vi "Vision Processing.vi"(7 "Image Size":T5=enum."320x240", 8 "error in (no error)":errorcluster, 11 "input cluster":T4={"Image Cal"="remote image 0000000011172DF4", "CameraDevRef"={"Camera Address"="USB 0", "CameraStatus"={"status"=FALSE, "code"=0, "source"=""}}, "Color"="remote image 000000001117C1BC", "Mask"="remote image 000000001106BF6C"}) -> ()   [LabVIEW 2016]
uses:
  Vision Support Code/Camera Types.ctl
  <vilib>/Rock Robotics/WPI/Camera/WPI_CameraImageSize.ctl
  <vilib>/vision/Image Controls.llb/IMAQ Image.ctl
  <vilib>/Rock Robotics/WPI/Camera/WPI_CameraDevRef.ctl
  Robot Global Data.vi
  <vilib>/Rock Robotics/Network Tables/NT Read Number.vi
  <vilib>/Rock Robotics/Network Tables/NT Read String.vi
  Vision Global.vi
  <vilib>/Rock Robotics/Network Tables/NT Write Number.vi
  <vilib>/Rock Robotics/Network Tables/NT Write String.vi
  <vilib>/vision/NI_Vision_Development_Module.lvlib
panel:
  out "LED Color":T1={"Hue"={30.0, 150.0}, "Sat"={0.0, 255.0}, "Val"={121.42857142857143, 255.0}} {"Hue" scale=0.0..255.0 scale format="%#_3g"}
  out "Size Limit %":dbl=0.04 format="%#_13g"
  out "Image":T2(plugin-control)
  out "error out":errorcluster
  out "loop ms":u32=37
  out "Calibration error":errorcluster
  in  "Display Original":bool=TRUE
  in  "Display Mask":bool=TRUE
  in  "Line Border":cluster{"Top":dbl, "Bottom":dbl}={"Top"=6.0, "Bottom"=1.0}
  in  "Use Calibration":bool
  in  "Color Mode":u16(ring)=3 items=["RGB", "HSL", "HSV", "HSI"]
  in  "Particles":dbl=2.0
  in  "Score Cutoff %":dbl=82.0
  in  "Camera Type":T6=enum."MS HD3000 square"
  out "Results":T7={"Distance (ft)"=0.0, "Score"=0.0, "Normalized"={"Center"={-1.0, 1.0}, "Rectangle"={"Numeric"=-1.0, "Numeric 2"=1.0, "Numeric 3"=-1.0, "Numeric 5"=1.0}}, "Pixels"={"Center"={0.0, 0.0}, "Rectangle"={"Numeric"=0.0, "Numeric 2"=0.0, "Numeric 3"=0.0, "Numeric 5"=0.0}}} {"Score" format="%#_3g"; "Pixels"."Rectangle"."Numeric 5" format="%#_3g"; "Pixels"."Rectangle"."Numeric 3" format="%#_3g"; "Pixels"."Rectangle"."Numeric 2" format="%#_3g"; "Pixels"."Rectangle"."Numeric" format="%#_3g"; "Normalized"."Rectangle"."Numeric 5" format="%#_2g"; "Normalized"."Rectangle"."Numeric 3" format="%#_2g"; "Normalized"."Rectangle"."Numeric 2" format="%#_2g"; "Normalized"."Rectangle"."Numeric" format="%#_2g"; "Normalized"."Center"."?" format="%#_3g"; "Normalized"."Center"."?" format="%#_3g"; "Distance (ft)" format="%#_3g"}
  out "Qualified Particles":i32
  # "This is now indicator"
  # "Legend:\n    Rectangle\n       Green - Good target, distance ft\n       Red - Bad target\n    Orange Text - Score in %"
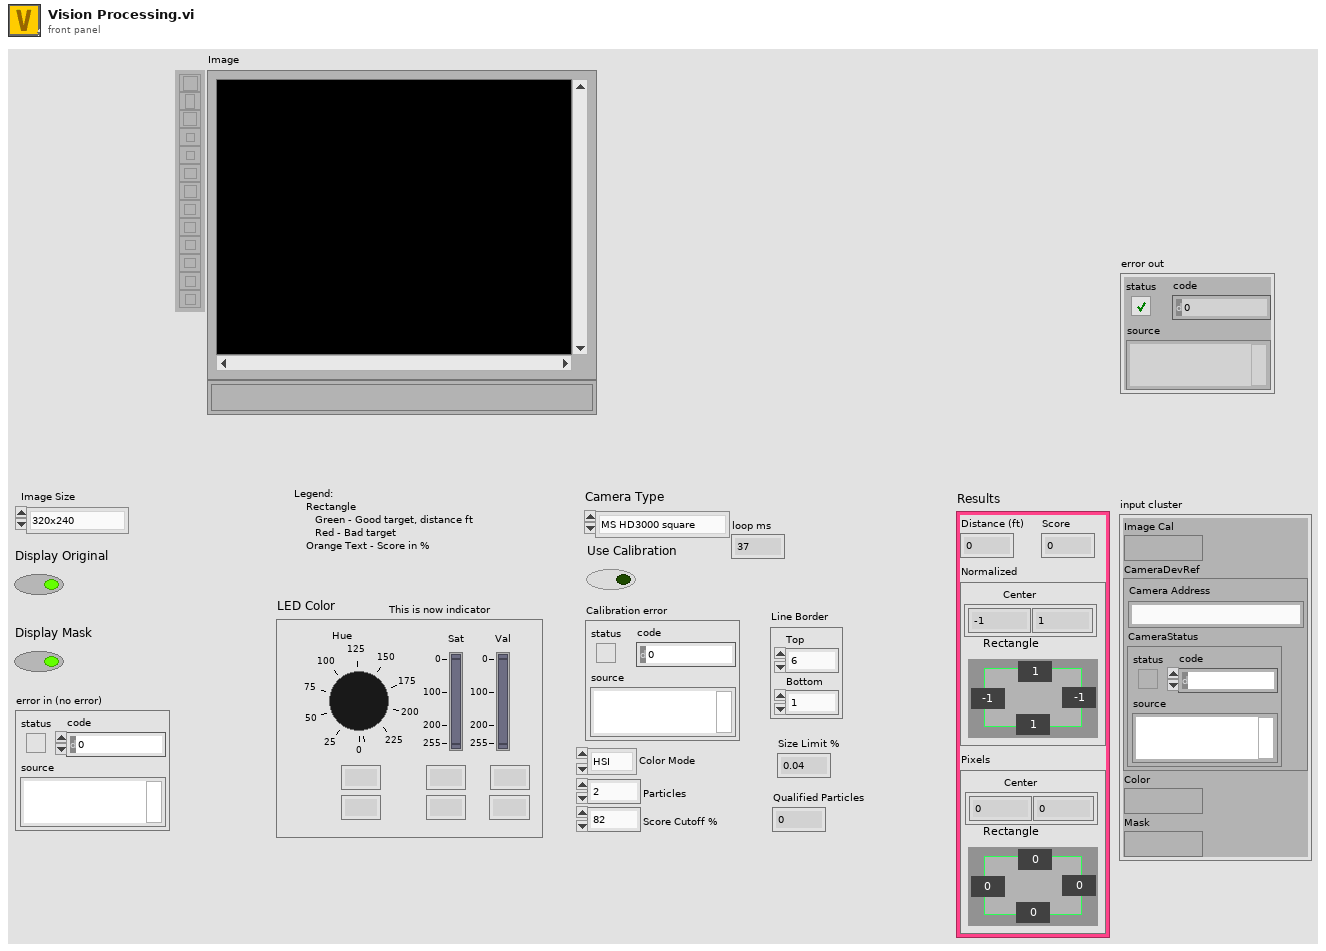
[diagram p1: front panel]
types:
  T1 = cluster{"Hue":cluster{dbl, dbl}, "Sat":cluster{dbl, dbl}, "Val":cluster{dbl, dbl}}
  T2 = typedef "IMAQ Image.ctl" = refnum<image>
  T3 = typedef "WPI_CameraDevRef.ctl" = cluster{"Camera Address":string, "CameraStatus":errorcluster}
  T4 = cluster{"Image Cal":T2, "CameraDevRef":T3, "Color":T2, "Mask":T2}
  T5 = typedef "WPI_CameraImageSize.ctl" = enum16{"640x480", "320x240", "160x120", "Custom"}
  T6 = typedef "Camera Types.ctl" = enum16{"206", "1011", "1013", "MS HD3000 square", "MS HD3000 640x480"}
  T7 = cluster{"Distance (ft)":dbl, "Score":dbl, "Normalized":cluster{"Center":cluster{dbl, dbl}, "Rectangle":cluster{"Numeric":dbl, "Numeric 2":dbl, "Numeric 3":dbl, "Numeric 5":dbl}}, "Pixels":cluster{"Center":cluster{dbl, dbl}, "Rectangle":cluster{"Numeric":dbl, "Numeric 2":dbl, "Numeric 3":dbl, "Numeric 5":dbl}}}
  T8 = typedef "Particle Parameters" = i32
  T9 = cluster{"Left":dbl, "Top":dbl, "Right":dbl, "Bottom":dbl}
  T10 = cluster{"Image out":T2, "Results":cluster{"Distance (ft)":dbl, "Score":dbl, "Normalized":cluster{"Center":cluster{dbl, dbl}, "Rectangle":cluster{"Numeric":dbl, "Numeric 2":dbl, "Numeric 3":dbl, "Numeric 5":dbl}}, "Pixels":cluster{"Center":cluster{dbl, dbl}, "Rectangle":cluster{"Numeric":dbl, "Numeric 2":dbl, "Numeric 3":dbl, "Numeric 5":dbl}}}, "Edges":cluster{"X":sgl, "Y":sgl}[]}
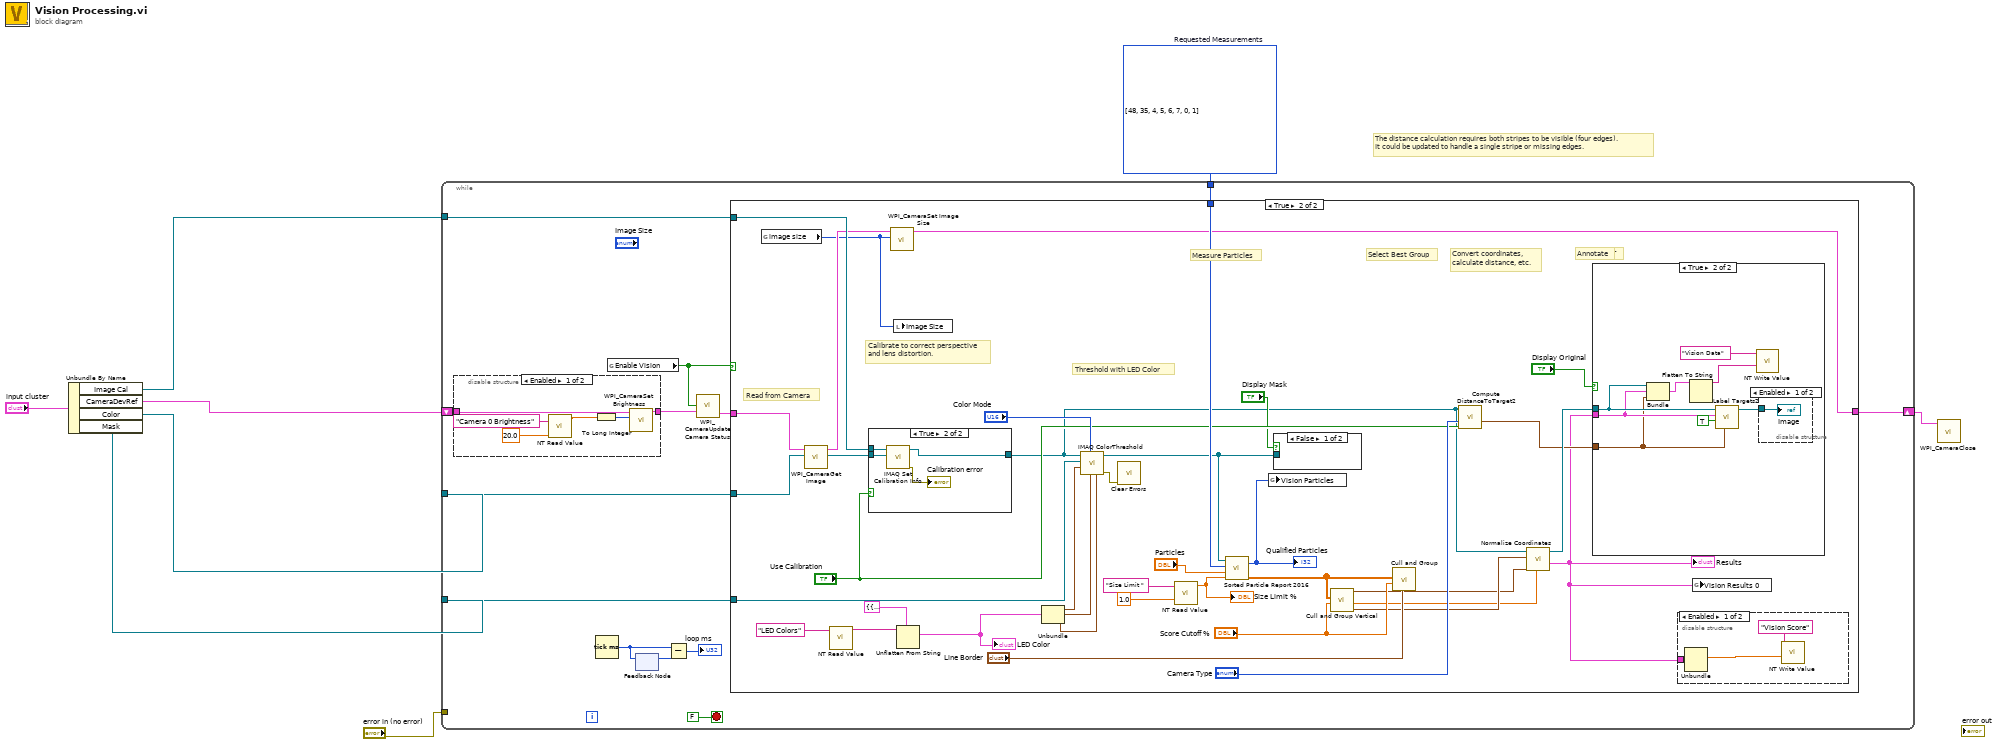
[diagram p0: block diagram]
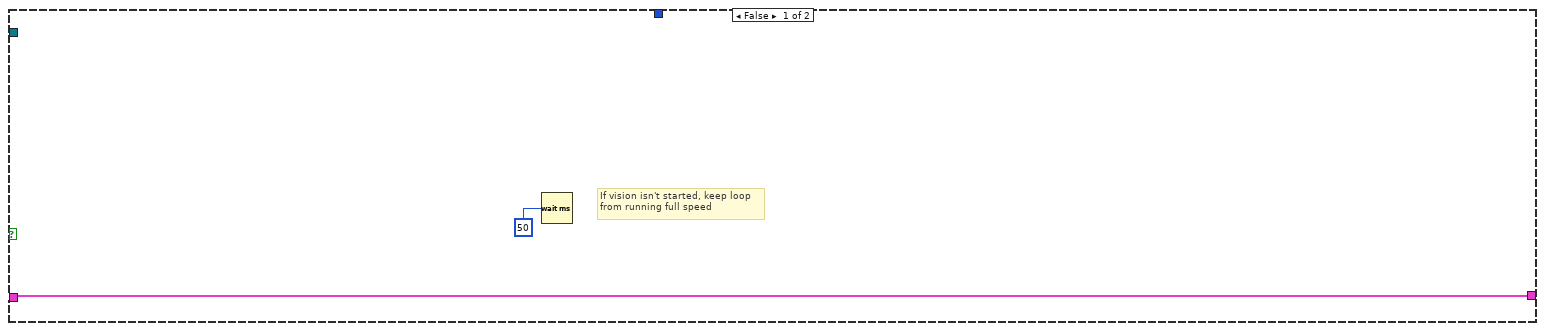
[diagram p3: hidden frame]
diagram:
  w7 = T8[] [48, 35, 4, 5, 6, 7, 0, 1] items=["Center of Mass X", "Center of Mass Y", "First Pixel X", "First Pixel Y", "Bounding Rect Left", "Bounding Rect Top", "Bounding Rect Right", "Bounding Rect Bottom", "Max Feret Diameter Start X", "Max Feret Diameter Start Y", "Max Feret Diameter End X", "Max Feret Diameter End Y", "Max Horiz. Segment Length Left", "Max Horiz. Segment Length Right", "Max Horiz. Segment Length Row", "-", "Bounding Rect Width", "Bounding Rect Height", "Bounding Rect Diagonal", "Perimeter", "Convex Hull Perimeter", "Holes' Perimeter", "Max Feret Diameter", "Equivalent Ellipse Major Axis", "Equivalent Ellipse Minor Axis", "Equivalent Ellipse Minor Axis (Feret)", "Equivalent Rect Long Side", "Equivalent Rect Short Side", "Equivalent Rect Diagonal", "Equivalent Rect Short Side (Feret)", "Average Horiz. Segment Length", "Average Vert. Segment Length", "Hydraulic Radius", "Waddel Disk Diameter", "-", "Area", "Holes' Area", "Particle & Holes' Area", "Convex Hull Area", "Image Area", "-", "Number of Holes", "Number of Horiz. Segments", "Number of Vert. Segments", "-", "Orientation", "Max Feret Diameter Orientation", "-", "% Area/Image Area", "% Area/(Particle & Holes' Area)", "Ratio of Equivalent Ellipse Axes", "Ratio of Equivalent Rect Sides", "-", "Elongation Factor", "Compactness Factor", "Heywood Circularity Factor", "Type Factor", "-", "Sum X", "Sum Y", "Sum XX", "Sum XY", "Sum YY", "Sum XXX", "Sum XXY", "Sum XYY", "Sum YYY", "-", "Moment of Inertia XX", "Moment of Inertia XY", "Moment of Inertia YY", "Moment of Inertia XXX", "Moment of Inertia XXY", "Moment of Inertia XYY", "Moment of Inertia YYY", "Norm. Moment of Inertia XX", "Norm. Moment of Inertia XY", "Norm. Moment of Inertia YY", "Norm. Moment of Inertia XXX", "Norm. Moment of Inertia XXY", "Norm. Moment of Inertia XYY", "Norm. Moment of Inertia YYY", "Hu Moment 1", "Hu Moment 2", "Hu Moment 3", "Hu Moment 4", "Hu Moment 5", "Hu Moment 6", "Hu Moment 7"]  # Requested Measurements
  # "The distance calculation requires both stripes to be visible (four edges).\nIt could be updated to handle a single stripe or missing edges."
  n1 = Unbundle By Name("input cluster") -> ("Image Cal"=w5:T2, "CameraDevRef"=w4:T3, "Color"=w6:T2, "Mask"=w8:T2)
  n2 = while {
    tunnel: w6 -> [w17]
    tunnel: w8 -> [w20]
    tunnel: w7 -> [w19]
    tunnel: w5 -> [w18]
    shift-right: [w16] -> w3
    shift-left: w4 -> [w10]
    tunnel: "error in (no error)" -> [_]
    stop <- FALSE stop-if-true
    n3 = disable-structure shown="Enabled" {
      disable-tunnel: w10 -> [w27 w28]
      disable-tunnel: [w26 w28] -> w9
      frame Enabled {
        n4 = call-poly <vilib>:"NT Read Value.vi"("Default Value"=20.0, "Name"="Camera 0 Brightness") -> ("Numeric"=w24:dbl)  [unwired: 8 in, 1 out]
        n5 = To Long Integer(number=w24) -> (32bit integer=w22:i32)
        n6 = call <vilib>:"WPI_CameraSet Brightness.vi"("Brightness"=w22, "CameraDevRef"=w27) -> ("CameraDevRef Out"=w26:T3)  [unwired: 1 in, 8 out]
      }
      frame Disabled {
      }
    }
    n7 = Tick Count (ms)() -> (millisecond timer value=w12:u32)
    n8 = global read "Robot Global Data.vi" "Enable Vision"() -> (w14:bool)
    n9 = feedback-in #1(w12) -> ()
    n10 = feedback #1() -> (w13:u32)  [unwired: 1 in]
    n11 = Subtract(x=w12, y=w13) -> (x-y=→"loop ms":u32)
    n12 = call <vilib>:"WPI_CameraUpdate Camera Status.vi"("CameraDevRef In"=w9, "Enable Vision"=w14) -> ("CameraDevRef Out"=w15:T3)  [unwired: 3 in]
    n13 = case shown="True" w14 {
      tunnel: w20 -> [_ w68]
      tunnel: w19 -> [_ w64]
      tunnel: w18 -> [_ w56]
      tunnel: w15 -> [w30 w53]
      tunnel: w17 -> [_ w52]
      tunnel: [w30 w47] -> w16
      frame False {
        # "If vision isn't started, keep loop\nfrom running full speed"
        n14 = Wait (ms)(milliseconds to wait=u32 50) -> ()  [unwired: 1 out]
      }
      frame True {
        # "Write to NT"
        # "Read from Camera"
        # "Calibrate to correct perspective\nand lens distortion."
        # "Measure Particles"
        # "Convert coordinates,\ncalculate distance, etc."
        # "Annotate"
        # "Select Best Group"
        # "Threshold with LED Color"
        n15 = global read "Robot Global Data.vi" "image size"() -> (w46:T5)
        n16 = call <vilib>:"WPI_CameraGet Image.vi"("Image"=w52, "CameraDevRef"=w53) -> ("Image Out"=w51:T2, "CameraDevRef Out"=w48:T3)  [unwired: 7 in, 1 out]
        n17 = call-poly <vilib>:"NT Read Value.vi"("Name"="LED Colors") -> ("String"=w37:string)  [unwired: 9 in, 1 out]
        n18 = case shown="True" "Use Calibration" {
          tunnel: [w81 w85] -> w42
          tunnel: w51 -> [w81 w84]
          tunnel: w56 -> [_ w83]
          frame False {
          }
          frame True {
            n19 = call "IMAQ Set Calibration Info"("Image Dst"=w84, "Image Src"=w83) -> ("error out"=→"Calibration error":errorcluster, "Calibrated Image"=w85:T2)  [unwired: 8 in]
          }
        }
        n20 = call <vilib>:"WPI_CameraSet Image Size.vi"("Image Size"=w46, "CameraDevRef"=w48) -> ("CameraDevRef Out"=w47:T3)  [unwired: 2 in, 7 out]
        n21 = local write "Image Size"(w46) -> ()
        n22 = Unflatten From String(type=T1 {"Hue"={100.0, 140.0}, "Sat"={0.0, 255.0}, "Val"={121.42857142857143, 255.0}} ("LED Color"), binary string=w37) -> (value=w34:T1)  [unwired: 3 in, 2 out]
        "LED Color" <- w34
        n23 = Unbundle(w34) -> ("Hue"=w67:cluster{dbl, dbl}, "Sat"=w66:cluster{dbl, dbl}, "Val"=w65:cluster{dbl, dbl})
        n24 = call "IMAQ ColorThreshold"("Blue or Luma or Val or Inten Range"=w65, "Green or Sat Range"=w66, "Color Mode"="Color Mode", "Red or Hue Range"=w67, "Image Dst"=w68, "Image Src"=w42) -> ("error out"=w63:errorcluster, "Image Dst Out"=w62:T2)  [unwired: 4 in]
        n25 = call <vilib>:"Clear Errors.vi"("error in (no error)"=w63) -> ()  [unwired: 5 in, 2 out]
        n26 = call-poly <vilib>:"NT Read Value.vi"("Default Value"=1.0, "Name"="Size Limit ") -> ("Numeric"=w31:dbl)  [unwired: 8 in, 1 out]
        "Size Limit %" <- w31
        n27 = call "Sorted Particle Report 2016.vi"("Min Area Size %"=w31, "Particle Count Limit"="Particles", "Pixel Measurements"=w64, "Image in"=w62) -> ("Sorted Data"=w44:dbl[][], "Particles"=w41:i32)
        "Qualified Particles" <- w41
        n28 = global write "Vision Global.vi" "Vision Particles"(w41) -> ()
        n29 = case shown="False" "Display Mask" {
          tunnel: w62 -> [_ _]
          frame False {
          }
          frame True {
          }
        }
        n30 = call "Cull and Group Vertical.vi"("Score Cutoff"="Score Cutoff %", "Sorted Data"=w44) -> ("Rect"=w40:T9, "Top Score"=w39:dbl, "Center"=w38:cluster{"X":dbl, "Y":dbl})  [unwired: 7 in]
        n31 = call "Cull and Group.vi"("Line Border"="Line Border", "Score Cutoff"="Score Cutoff %", "Sorted Data"=w44) -> ()  [unwired: 5 in, 4 out]
        n32 = call "Compute DistanceToTarget2.vi"("Calibrated"="Use Calibration", "Camera Type"="Camera Type", "Image Src"=w42) -> ("Edges"=w57:cluster{"X":sgl, "Y":sgl}[])  [unwired: 6 in, 2 out]
        n33 = call "Normalize Coordinates.vi"("Score"=w39, "Center"=w38, "Bounding box"=w40, "Image in"=w42) -> ("Results"=w45:T7, "Image out"=w60:T2)  [unwired: 6 in]
        "Results" <- w45
        n34 = case shown="True" "Display Original" {
          tunnel: w60 -> [_ w77]
          tunnel: w45 -> [_ w76]
          tunnel: w57 -> [_ w75]
          frame False {
          }
          frame True {
            n35 = Bundle("Image out"=w77, "Results"=w76, "Edges"=w75) -> (w74:T10)  [unwired: 1 in]
            n36 = Flatten To String(anything=w74) -> (data string=w73:string)  [unwired: 3 in, 2 out]
            n37 = call "Label Targets2.vi"("Edges"=w75, "Annotate"=TRUE, "Results"=w76, "Image in"=w77) -> ("Image out"=w79:T2)  [unwired: 7 in]
            n38 = call-poly <vilib>:"NT Write Value.vi"("String"=w73, "Name"="Vision Data") -> ()  [unwired: 9 in, 1 out]
            n39 = disable-structure shown="Enabled" {
              disable-tunnel: w79 -> [w80 _]
              frame Enabled {
                "Image" <- w80
              }
              frame Disabled {
              }
            }
          }
        }
        n40 = disable-structure shown="Enabled" {
          disable-tunnel: w45 -> [w71 _]
          frame Enabled {
            n41 = Unbundle(w71) -> ("Score"=w70:dbl)  [unwired: 3 out]
            n42 = call-poly <vilib>:"NT Write Value.vi"("Numeric"=w70, "Name"="Vision Score") -> ()  [unwired: 9 in, 1 out]
          }
          frame Disabled {
          }
        }
        n43 = global write "Vision Global.vi" "Vision Results 0"(w45) -> ()
      }
    }
  }
  n44 = call <vilib>:"WPI_CameraClose.vi"("CameraDevRef"=w3) -> ()  [unwired: 1 in, 10 out]
